vi "SetHight.vi"(8 "error in (no error)":errorcluster, 10 "Hight":i16, 11 "Triangle in":refnum<class "Losange.lvclass">) -> (0 "error out":errorcluster, 3 "Triangle out":refnum<class "Losange.lvclass">)   [LabVIEW 2021, in "Picture2D.lvlib" / "Losange.lvclass"]
uses:
  Losange.lvclass
  Losange.lvclass/Losange.ctl
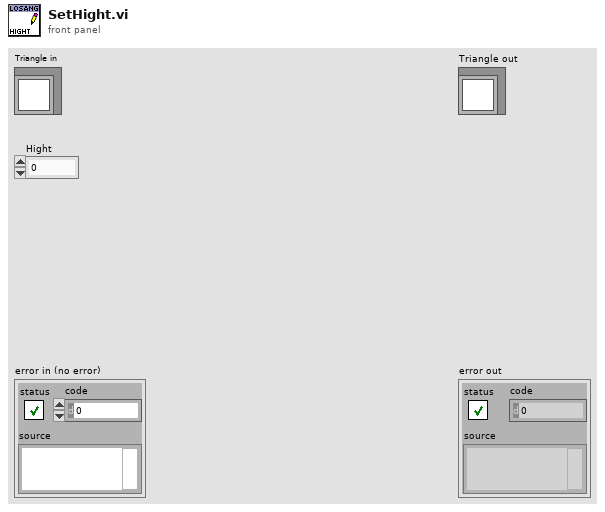
[diagram p1: front panel]
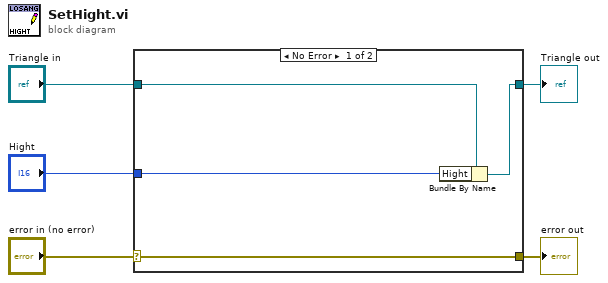
[diagram p0: block diagram]
diagram:
  n1 = case shown="No Error" "error in (no error)" {
    selector: "error in (no error)" -> [w9 w10]
    tunnel: [w9 w10] -> w4
    tunnel: [w7 w11] -> w2
    tunnel: "Triangle in" -> [w8 w11]
    tunnel: "Hight" -> [w6 _]
    frame No Error {
      n2 = Bundle By Name(cluster=w8, "Hight"=w6) -> (w7:refnum<class "Losange.lvclass">)
    }
    frame Error {
    }
  }
  "error out" <- w4
  "Triangle out" <- w2
